vi "mass_flow_rate.vi"(1 "Density":dbl[](array[numeric]), 2 "dP Pa":dbl[](array[numeric])) -> (0 "Mass Flow Rate [g/s] Array":dbl[](array[numeric]))   [LabVIEW 2017]
uses:
  Sensor Translation/sensor_translation.lvlib
  Sensor Translation/pressure_unit_converter.vi
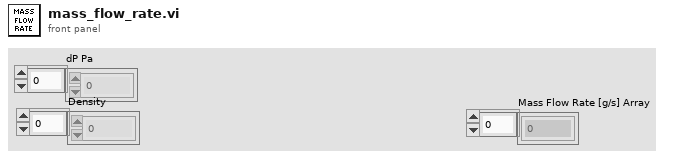
[diagram p1: front panel]
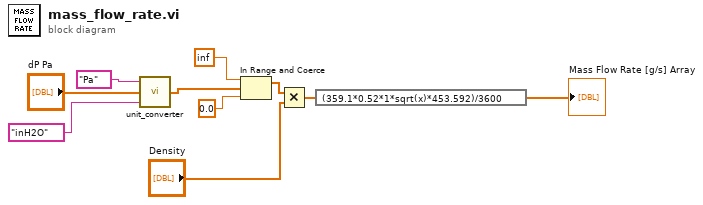
[diagram p0: block diagram]
diagram:
  n1 = call-poly "unit_converter.vi"("Output Unit"="inH2O", "Input"="dP Pa", "Input Unit"="Pa") -> ("Output"=w2:dbl[])
  n2 = In Range and Coerce(upper limit=inf, x=w2, lower limit=0.0 ("upper limit")) -> (coerced(x)=w4:dbl[])  [unwired: 1 out]
  n3 = Multiply(x=w4, y="Density") -> (x*y=w9:dbl[])
  n4 = expression code="(359.1*0.52*1*sqrt(x)*453.592)/3600"(w9) -> (→"Mass Flow Rate [g/s] Array":dbl[])
